vi "Describe Comparison of Arrays.vi"(8 "error in (no error)":errorcluster, 9 "Actual":variant[](array[variant]), 10 "Expected":variant[](array[variant])) -> (0 "error out":errorcluster, 2 "Description":string)   [LabVIEW 2020, in "LUnit Test Case.lvclass"]
uses:
  LUnit Test Case.lvclass
  <vilib>/Utility/Data Type/Get Type Information.vi
  <vilib>/Utility/LVClass/Get LV Class Name.vi
  LUnit Test Case.lvclass/LUnit Test Case.ctl
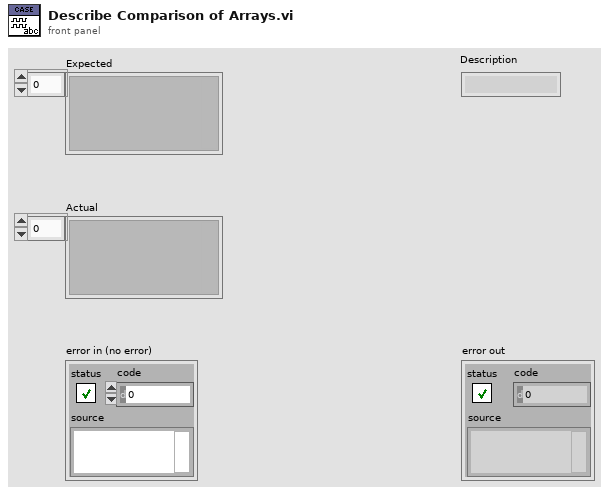
[diagram p1: front panel]
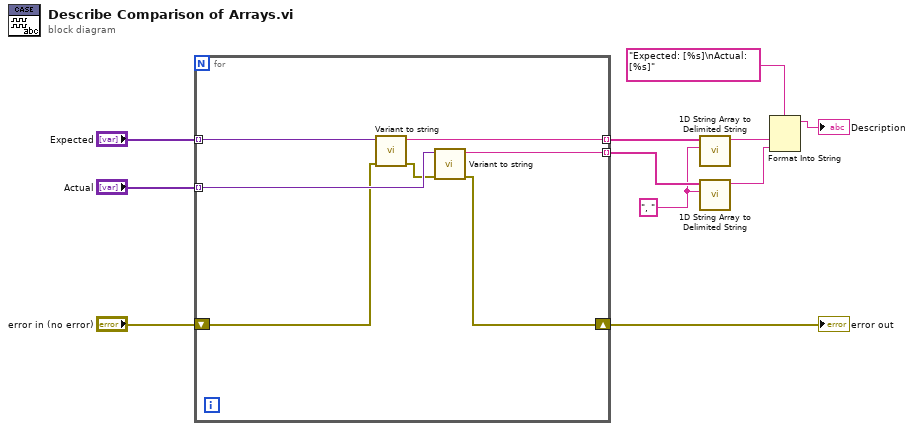
[diagram p0: block diagram]
diagram:
  w1 = ", " ("delimiter")
  n1 = for {
    tunnel: "Expected" -> [w18] mode=indexing
    tunnel: "Actual" -> [w17] mode=indexing
    shift-right: [w15] -> w8
    shift-left: "error in (no error)" -> [w16]
    tunnel: [w13] -> w4 mode=indexing
    tunnel: [w12] -> w5 mode=indexing
    n2 = call "Variant to string.vi"("error in (no error)"=w16, "Variant"=w18) -> ("error out"=w14:errorcluster, "String"=w13:string)  [unwired: 8 in]
    n3 = call "Variant to string.vi"("error in (no error)"=w14, "Variant"=w17) -> ("error out"=w15:errorcluster, "String"=w12:string)  [unwired: 8 in]
  }
  "error out" <- w8
  n4 = call <vilib>:"1D String Array to Delimited String.vi"("delimiter"=w1, "string array"=w4) -> ("delimited string"=w3:string)  [unwired: 9 in]
  n5 = call <vilib>:"1D String Array to Delimited String.vi"("delimiter"=w1, "string array"=w5) -> ("delimited string"=w2:string)  [unwired: 9 in]
  n6 = Format Into String(format string="Expected: [%s]\nActual:   [%s]", w3, w2) -> (resulting string=→"Description":string)  [unwired: 2 in, 1 out]
